vi "Send Notification.vi"(4 "Paras In 2":variant, 6 "Paras In":variant, 7 "Timeout":i32=-1, 8 "error in (no error)":errorcluster, 9 "Notification In":variant, 10 "Mail Strategy":refnum<class "Mail Strategy.lvclass">, 11 "Notifier Controller in":refnum<class "Notifier Controller.lvclass">) -> (0 "error out":errorcluster, 3 "Notifier Controller out":refnum<class "Notifier Controller.lvclass">)   [LabVIEW 2024, in "Notifier Controller.lvclass"]
uses:
  Notifier Controller.lvclass
  Messenger/Mail Strategy/Mail Strategy.lvclass
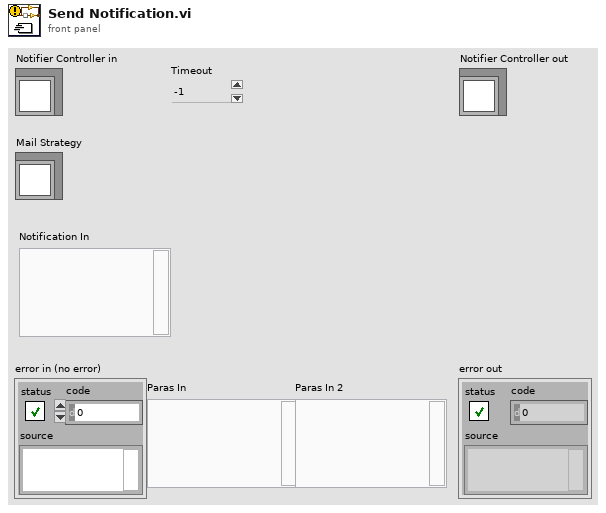
[diagram p1: front panel]
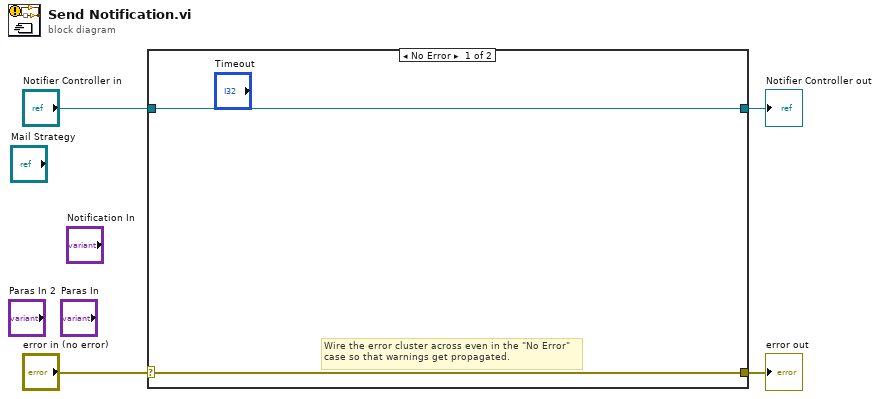
[diagram p0: block diagram]
diagram:
  n1 = case shown="No Error" "error in (no error)" {
    selector: "error in (no error)" -> [w5 w8]
    tunnel: [w5 w8] -> w3
    tunnel: [w6 w7] -> w1
    tunnel: "Notifier Controller in" -> [w6 w7]
    frame No Error {
      # "Wire the error cluster across even in the \"No Error\"\ncase so that warnings get propagated."
    }
    frame Error {
    }
  }
  "error out" <- w3
  "Notifier Controller out" <- w1
